vi "sub_getArrayValues.vi"(11 "controls":refnum<vi>[](array[refnum])) -> (3 "array":string[](array[string]))   [LabVIEW 2018]
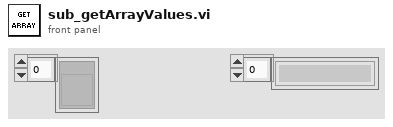
[diagram p1: front panel]
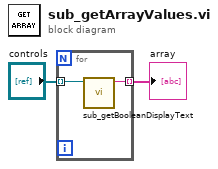
[diagram p0: block diagram]
diagram:
  n1 = for {
    tunnel: "controls" -> [w4] mode=indexing
    tunnel: [w3] -> w1 mode=indexing
    n2 = call "sub_getBooleanDisplayText.vi"(11:w4) -> ("True Label"=w3:string)  [unwired: 10 in]
  }
  "array" <- w1
